vi "Read Buffer Data.vi"(8 "error in (no error)":errorcluster, 9 "Data Index (1)":i32=1, 10 "Reading Buffer (smua.nvbuffer1)":string="smua.nvbuffer1", 11 "VISA resource name":refnum<visa-resource-name>) -> (0 "error out":errorcluster, 1 "Data Source":dbl, 2 "Data Value":dbl, 3 "VISA resource name out":refnum<visa-resource-name>, 5 "Data Timestamp":timestamp)   [LabVIEW 2019, in "Keithley 2600 Series.lvlib"]
doc: "Returns the reading, source value and timestamp stored in a specified reading buffer."
uses:
  Keithley 2600 Series.lvlib
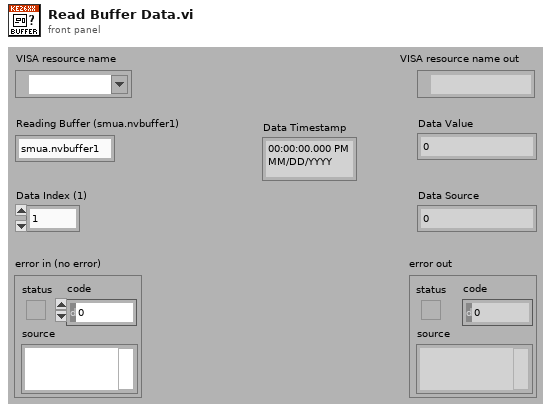
[diagram p1: front panel]
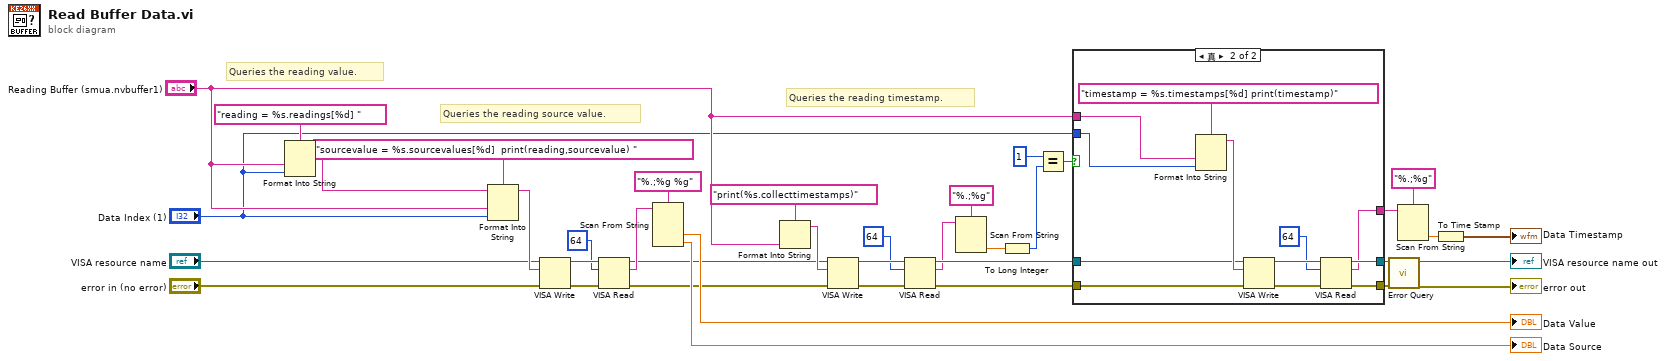
[diagram p0: block diagram]
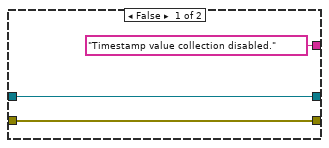
[diagram p2: hidden frame]
diagram:
  # "Queries the reading timestamp."
  # "Queries the reading source value."
  # "Queries the reading value."
  n1 = Format Into String(format string="reading = %s.readings[%d] ", "Reading Buffer (smua.nvbuffer1)", "Data Index (1)") -> (resulting string=w25:string)  [unwired: 2 in, 1 out]
  n2 = Format Into String(format string="sourcevalue = %s.sourcevalues[%d]  print(reading,sourcevalue) ", initial string=w25, "Reading Buffer (smua.nvbuffer1)", "Data Index (1)") -> (resulting string=w36:string)  [unwired: 1 in, 1 out]
  n3 = VISA Write(VISA resource name="VISA resource name", write buffer=w36, error in (no error)="error in (no error)") -> (VISA resource name out=w31:refnum<visa-resource-name>, error out=w30:errorcluster)  [unwired: 1 out]
  n4 = VISA Read(VISA resource name=w31, byte count=u32 64, error in (no error)=w30) -> (VISA resource name out=w19:refnum<visa-resource-name>, read buffer=w28:string, error out=w18:errorcluster)  [unwired: 1 out]
  n5 = Scan From String(format string="%.;%g %g", input string=w28) -> (output 1=→"Data Value":dbl, output 2=→"Data Source":dbl)  [unwired: 4 in, 3 out]
  n6 = Format Into String(format string="print(%s.collecttimestamps)", "Reading Buffer (smua.nvbuffer1)") -> (resulting string=w20:string)  [unwired: 2 in, 1 out]
  n7 = VISA Write(VISA resource name=w19, write buffer=w20, error in (no error)=w18) -> (VISA resource name out=w23:refnum<visa-resource-name>, error out=w22:errorcluster)  [unwired: 1 out]
  n8 = VISA Read(VISA resource name=w23, byte count=u32 64, error in (no error)=w22) -> (VISA resource name out=w16:refnum<visa-resource-name>, read buffer=w9:string, error out=w15:errorcluster)  [unwired: 1 out]
  n9 = Scan From String(format string="%.;%g", input string=w9) -> (output 1=w7:dbl)  [unwired: 3 in, 3 out]
  n10 = To Long Integer(number=w7) -> (32bit integer=w6:i32)
  n11 = Equal?(x=1, y=w6) -> (x = y?=w14:bool)
  n12 = case shown="真" w14 {
    tunnel: w16 -> [w41 w48]
    tunnel: w15 -> [w40 w47]
    tunnel: [w41 w46] -> w13
    tunnel: [w40 w45] -> w12
    tunnel: ["Timestamp value collection disabled." ("read buffer") w44] -> w4
    tunnel: "Reading Buffer (smua.nvbuffer1)" -> [_ w43]
    tunnel: "Data Index (1)" -> [_ w42]
    frame False {
    }
    frame True {
      n13 = Format Into String(format string="timestamp = %s.timestamps[%d] print(timestamp)", w43, w42) -> (resulting string=w50:string)  [unwired: 2 in, 1 out]
      n14 = VISA Write(VISA resource name=w48, write buffer=w50, error in (no error)=w47) -> (VISA resource name out=w53:refnum<visa-resource-name>, error out=w52:errorcluster)  [unwired: 1 out]
      n15 = VISA Read(VISA resource name=w53, byte count=u32 64, error in (no error)=w52) -> (VISA resource name out=w46:refnum<visa-resource-name>, read buffer=w44:string, error out=w45:errorcluster)  [unwired: 1 out]
    }
  }
  n16 = call "Error Query.vi"("error in (no error)"=w12, "VISA resource name"=w13) -> ("error out"=→"error out":errorcluster, "VISA resource name out"=→"VISA resource name out":refnum<visa-resource-name>)  [unwired: 6 in, 2 out]
  n17 = Scan From String(format string="%.;%g", input string=w4) -> (output 1=w3:dbl)  [unwired: 3 in, 3 out]
  n18 = To Time Stamp(1:w3) -> (0:→"Data Timestamp":timestamp)
